vi "cmd_list.vi"(11 "CMD":T2=enum."MEMORY AREA READ") -> (3 "cmd":T1, 5 "item":string)   [LabVIEW 2020, in "FINS TCP.lvlib"]
uses:
  FINS TCP.lvlib
  FINS CMD item.ctl
  FINS CMD.ctl
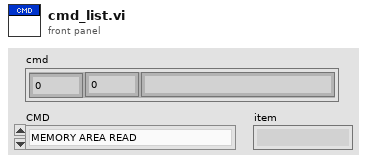
[diagram p1: front panel]
types:
  T1 = typedef "FINS TCP.lvlib/FINS CMD.ctl" = cluster{"MR":u8, "SR":u8, "name":string}
  T2 = typedef "FINS TCP.lvlib/FINS CMD item.ctl" = enum16{"FINS_UNKNOWN", "FINS_SETUP", "MEMORY AREA READ", "MEMORY AREA WRITE", "MEMORY AREA FILL", "MULTIPLE MEMORY AREA READ", "MEMORY AREA TRANSFER", "PARAMETER AREA READ", "PARAMETER AREA WRITE", "PARAMETER AREA CLEAR", "PROGRAM AREA PROTECT", "PROGRAM AREA PROTECT CLEAR", "PROGRAM AREA READ", "PROGRAM AREA WRITE", "PROGRAM AREA CLEAR", "RUN", "STOP", "CONTROLLER DATA READ", "CONNECTION DATA READ", "CONTROLLER STATUS READ", "CYCLE TIME READ", "CLOCK READ", "CLOCK WRITE", "MESSAGE READ", "MESSAGE CLEAR", "FAL/FALS READ", "ACCESS RIGHT ACQUIRE", "ACCESS RIGHT FORCED ACQUIRE", "ACCESS RIGHT RELEASE", "ERROR CLEAR", "ERROR LOG READ", "ERROR LOG CLEAR", "FILE NAME READ", "SINGLE FILE READ", "SINGLE FILE WRITE", "MEMORY CARD FORMAT", "FILE DELETE", "VOLUME LABEL CREATE/DELETE", "FILE COPY", "FILE NAME CHANGE", "FILE DATA CHECK", "MEMORY AREA FILE TRANSFER", "PARAMETER AREA FILE TRANSFER", "PROGRAM AREA FILE TRANSFER", "FORCED SET/RESET", "FORCED SET/RESET CANCEL"}
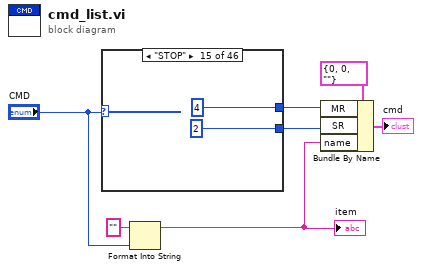
[diagram p0: block diagram]
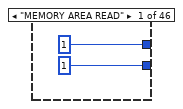
[diagram p2: hidden frame]
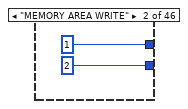
[diagram p3: hidden frame]
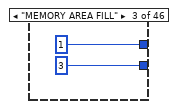
[diagram p4: hidden frame]
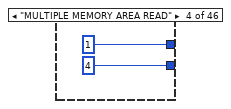
[diagram p5: hidden frame]
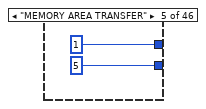
[diagram p6: hidden frame]
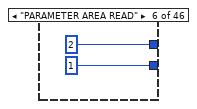
[diagram p7: hidden frame]
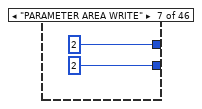
[diagram p8: hidden frame]
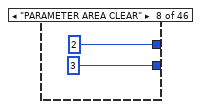
[diagram p9: hidden frame]
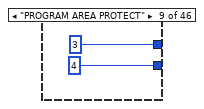
[diagram p10: hidden frame]
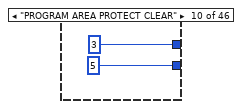
[diagram p11: hidden frame]
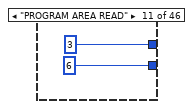
[diagram p12: hidden frame]
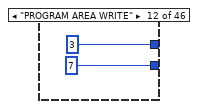
[diagram p13: hidden frame]
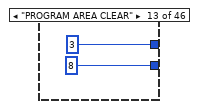
[diagram p14: hidden frame]
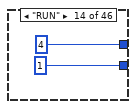
[diagram p15: hidden frame]
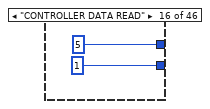
[diagram p16: hidden frame]
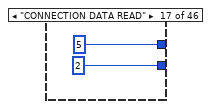
[diagram p17: hidden frame]
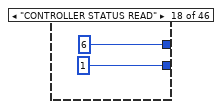
[diagram p18: hidden frame]
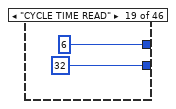
[diagram p19: hidden frame]
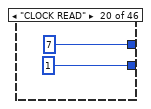
[diagram p20: hidden frame]
diagram:
  n1 = case shown="\"STOP\"" "CMD" {
    tunnel: [u8 1 ("MR") u8 1 ("MR") u8 1 ("MR") u8 1 ("MR") u8 1 ("MR") u8 2 ("MR") u8 2 ("MR") u8 2 ("MR") u8 3 ("MR") u8 3 ("MR") u8 3 ("MR") u8 3 ("MR") u8 3 ("MR") u8 4 ("MR") u8 4 ("MR") u8 5 ("MR") u8 5 ("MR") u8 6 ("MR") u8 6 ("MR") u8 7 ("MR") u8 7 ("MR") u8 9 ("MR") u8 9 ("MR") u8 9 ("MR") u8 12 ("MR") u8 12 ("MR") u8 12 ("MR") u8 33 ("MR") u8 33 ("MR") u8 33 ("MR") u8 34 ("MR") u8 34 ("MR") u8 34 ("MR") u8 34 ("MR") u8 34 ("MR") u8 34 ("MR") u8 34 ("MR") u8 34 ("MR") u8 34 ("MR") u8 34 ("MR") u8 34 ("MR") u8 34 ("MR") u8 35 ("MR") u8 35 ("MR") u8 0 ("MR") u8 0 ("MR")] -> w3
    tunnel: [u8 1 ("MR") u8 2 ("MR") u8 3 ("MR") u8 4 ("MR") u8 5 ("MR") u8 1 ("MR") u8 2 ("MR") u8 3 ("MR") u8 4 ("MR") u8 5 ("MR") u8 6 ("MR") u8 7 ("MR") u8 8 ("MR") u8 1 ("MR") u8 2 ("MR") u8 1 ("MR") u8 2 ("MR") u8 1 ("MR") u8 32 ("MR") u8 1 ("MR") u8 2 ("MR") u8 32 ("MR") u8 32 ("MR") u8 32 ("MR") u8 1 ("MR") u8 2 ("MR") u8 3 ("MR") u8 1 ("MR") u8 2 ("MR") u8 3 ("MR") u8 1 ("MR") u8 2 ("MR") u8 3 ("MR") u8 4 ("MR") u8 5 ("MR") u8 6 ("MR") u8 7 ("MR") u8 8 ("MR") u8 9 ("MR") u8 10 ("MR") u8 11 ("MR") u8 12 ("MR") u8 1 ("MR") u8 2 ("MR") u8 0 ("MR") u8 0 ("MR")] -> w2
    frame "MEMORY AREA READ" {
    }
    frame "MEMORY AREA WRITE" {
    }
    frame "MEMORY AREA FILL" {
    }
    frame "MULTIPLE MEMORY AREA READ" {
    }
    frame "MEMORY AREA TRANSFER" {
    }
    frame "PARAMETER AREA READ" {
    }
    frame "PARAMETER AREA WRITE" {
    }
    frame "PARAMETER AREA CLEAR" {
    }
    frame "PROGRAM AREA PROTECT" {
    }
    frame "PROGRAM AREA PROTECT CLEAR" {
    }
    frame "PROGRAM AREA READ" {
    }
    frame "PROGRAM AREA WRITE" {
    }
    frame "PROGRAM AREA CLEAR" {
    }
    frame "RUN" {
    }
    frame "STOP" {
    }
    frame "CONTROLLER DATA READ" {
    }
    frame "CONNECTION DATA READ" {
    }
    frame "CONTROLLER STATUS READ" {
    }
    frame "CYCLE TIME READ" {
    }
    frame "CLOCK READ" {
    }
    frame "CLOCK WRITE" {
    }
    frame "MESSAGE READ" {
    }
    frame "MESSAGE CLEAR" {
    }
    frame "FAL/FALS READ" {
    }
    frame "ACCESS RIGHT ACQUIRE" {
    }
    frame "ACCESS RIGHT FORCED ACQUIRE" {
    }
    frame "ACCESS RIGHT RELEASE" {
    }
    frame "ERROR CLEAR" {
    }
    frame "ERROR LOG READ" {
    }
    frame "ERROR LOG CLEAR" {
    }
    frame "FILE NAME READ" {
    }
    frame "SINGLE FILE READ" {
    }
    frame "SINGLE FILE WRITE" {
    }
    frame "MEMORY CARD FORMAT" {
    }
    frame "FILE DELETE" {
    }
    frame "VOLUME LABEL CREATE/DELETE" {
    }
    frame "FILE COPY" {
    }
    frame "FILE NAME CHANGE" {
    }
    frame "FILE DATA CHECK" {
    }
    frame "MEMORY AREA FILE TRANSFER" {
    }
    frame "PARAMETER AREA FILE TRANSFER" {
    }
    frame "PROGRAM AREA FILE TRANSFER" {
    }
    frame "FORCED SET/RESET" {
    }
    frame "FORCED SET/RESET CANCEL" {
    }
    frame "FINS_SETUP" {
    }
    frame "FINS_UNKNOWN", Default {
    }
  }
  n2 = Format Into String(initial string="", "CMD") -> (resulting string=w4:string)  [unwired: 2 in, 1 out]
  "item" <- w4
  n3 = Bundle By Name(cluster=T1 {"MR"=0, "SR"=0, "name"=""} ("FINS CMD"), "MR"=w3, "SR"=w2, "name"=w4) -> (→"cmd":T1)
